vi "Pet Watchdog 2.vi"(8 "error in (no error)":errorcluster, 11 "FPGA VI Reference Out":refnum<k20>) -> (0 "error out":errorcluster, 3 "FPGA VI Reference Out 2":refnum<k20>)   [LabVIEW 2015]
uses:
  RT/RT Global References.vi
  <vilib>/Utility/error.llb/Error Cluster From Error Code.vi
  <vilib>/rvi/errors/niLvFpgaAdjustHostInterfaceError.vi
  <vilib>/rvi/interface/nirviReadWriteControl/nirviReadWriteControl.xnode
  NiFpgaLv.dll
  <vilib>/rvi/interface/Simulation/niFpgaSimulationCallBeginRW.vi
  <vilib>/Utility/Variable/NI_VariableUtilities.lvlib
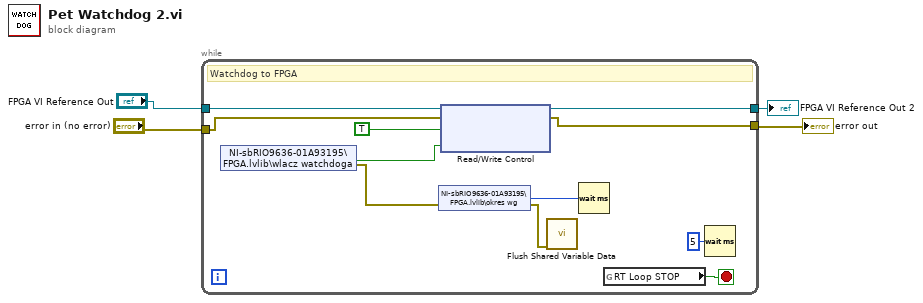
[diagram p0: block diagram]
diagram:
  n1 = while {
    tunnel: "FPGA VI Reference Out" -> [w15]
    tunnel: "error in (no error)" -> [w10]
    tunnel: [w9] -> w1
    tunnel: [w8] -> w3
    stop <- w6 stop-if-true
    # "Watchdog to FPGA"
    n2 = shared-variable "NI-sbRIO9636-01A93195\\FPGA.lvlib\\wlacz watchdoga"() -> (w12:bool, error out=w7:errorcluster)  [unwired: 1 in]
    n3 = shared-variable "NI-sbRIO9636-01A93195\\FPGA.lvlib\\okres wg"(error in=w7) -> (w13:u32, error out=w5:errorcluster)
    n4 = xnode "Read/Write Control"("FPGA VI Reference In"=w15, "error in"=w10, "watchdog"=TRUE, "wlacz watchdoga"=w12) -> ("FPGA VI Reference Out"=w9:refnum<k20>, "error out"=w8:errorcluster)
    n5 = call <vilib>:"Flush Shared Variable Data.vi"("error in (no error)"=w5) -> ()  [unwired: 10 in, 1 out]
    n6 = Wait (ms)(milliseconds to wait=w13) -> ()  [unwired: 1 out]
    n7 = global read "RT Global References.vi" "RT Loop STOP"() -> (w6:bool)
    n8 = Wait (ms)(milliseconds to wait=u32 5) -> ()  [unwired: 1 out]
  }
  "error out" <- w3
  "FPGA VI Reference Out 2" <- w1
